vi "Find first true boolean.vi"(0 "Boolean Array IN":bool[](array[boolean])) -> (3 "Index of first (T)":i32, 4 "True found?":bool)   [LabVIEW 2013]
doc: "Given a boolean array, this vi will return the index of the first boolean light that is on. If no lights are on, the returned value is 0."
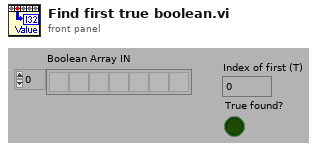
[diagram p1: front panel]
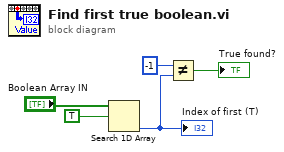
[diagram p0: block diagram]
diagram:
  n1 = Search 1D Array(1D array="Boolean Array IN", element=TRUE) -> (index of element=w3:i32)  [unwired: 1 out]
  "Index of first (T)" <- w3
  n2 = Not Equal?(x=-1, y=w3) -> (x != y?=→"True found?":bool)
